vi "tearDown.vi"(8 "error in (no error)":errorcluster, 11 "reference in":refnum<class "Add and Remove Test.lvclass">) -> (0 "error out":errorcluster, 3 "reference out":refnum<class "Add and Remove Test.lvclass">)   [LabVIEW 2019, in "Add and Remove Test.lvclass"]
doc: "tearDown runs after the test method has completed. Use this method to clean up any operations or references that were opened by setUp or the test method. Unit tests should be independent of other unit tests so this VI should ensure that the next test can run in a 'clean' test environment."
uses:
  Add and Remove Test.lvclass
  Add and Remove Test.lvclass/Add and Remove Test.ctl
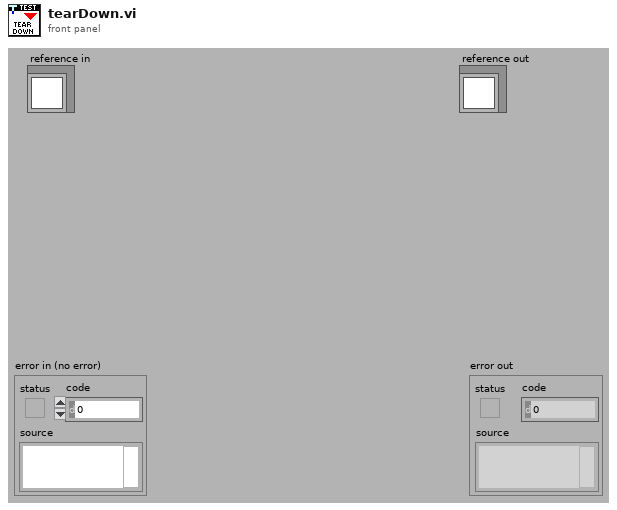
[diagram p1: front panel]
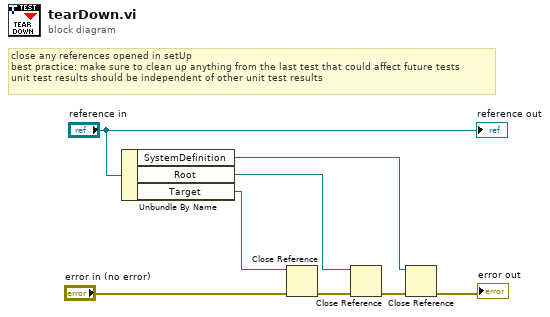
[diagram p0: block diagram]
diagram:
  # "close any references opened in setUp\nbest practice: make sure to clean up anything from the last test that could affect future tests\nunit test results should be independent of other unit test results"
  n1 = Unbundle By Name("reference in") -> ("SystemDefinition"=w4:refnum<k24>, "Root"=w6:refnum<k24>, "Target"=w8:refnum<k24>)
  n2 = Close Reference(reference=w8, error in (no error)="error in (no error)") -> (error out=w7:errorcluster)
  n3 = Close Reference(reference=w6, error in (no error)=w7) -> (error out=w5:errorcluster)
  n4 = Close Reference(reference=w4, error in (no error)=w5) -> (error out=→"error out":errorcluster)
  "reference out" <- "reference in"
